vi "OTF_subtraction.vi"(0 "Buffer Length":i32, 5 "Buffer":u32[](array[numeric]), 7 "Cluster In":T1 {"Coincidence Window" format="%#_13g"; "Delay12" format="%#_13g"; "Delay02" format="%#_13g"; "Delay01" format="%#_13g"}, 12 "ofl":u64) -> (3 "ofl out":u64, 8 "output cluster":T1 {"Coincidence Window" format="%#_13g"; "Delay12" format="%#_13g"; "Delay02" format="%#_13g"; "Delay01" format="%#_13g"})   [LabVIEW 2023]
uses:
  Get_Delays_Ctrl.ctl
panel:
  out "Delay02":dbl
  out "Delay12":dbl
  out "Trues":dbl
  out "Delay01":dbl
  out "Coincidence Triggers":u64
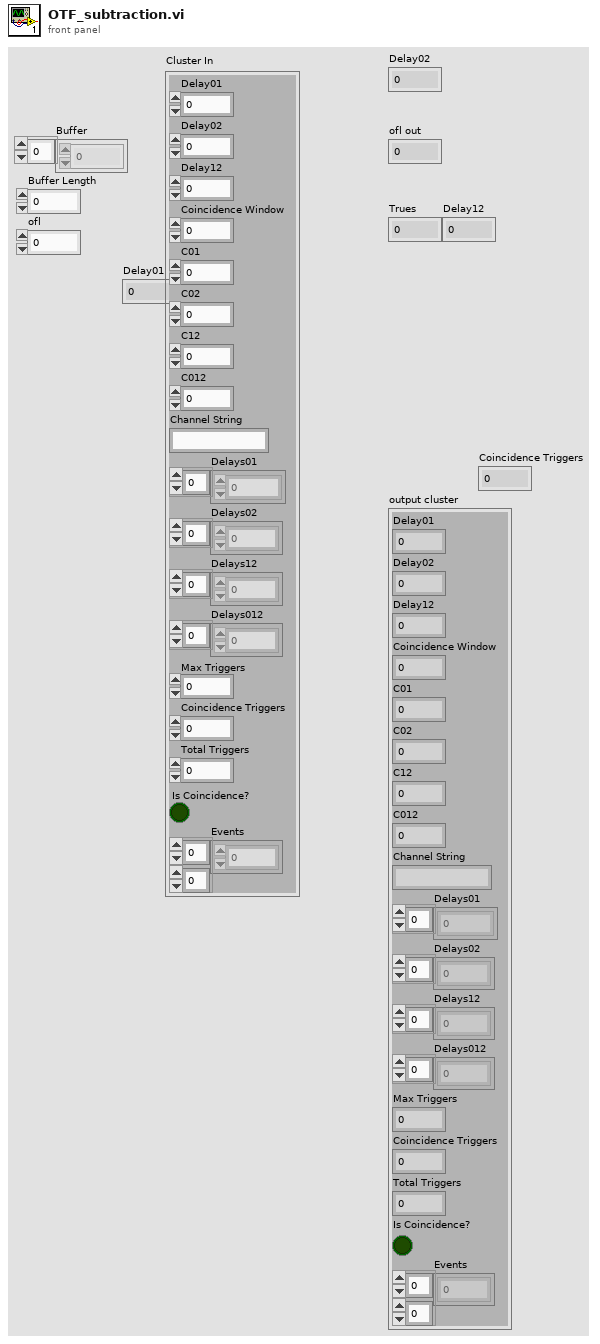
[diagram p1: front panel]
types:
  T1 = typedef "Get_Delays_Ctrl.ctl" = cluster{"Delay01":dbl, "Delay02":dbl, "Delay12":dbl, "Coincidence Window":dbl, "C01":u32, "C02":u32, "C12":u32, "C012":u32, "Channel String":string, "Delays01":sgl[], "Delays02":dbl[], "Delays12":dbl[], "Delays012":dbl[], "Max Triggers":i32, "Coincidence Triggers":i32, "Total Triggers":i32, "Is Coincidence?":bool, "Events":u64[][]}
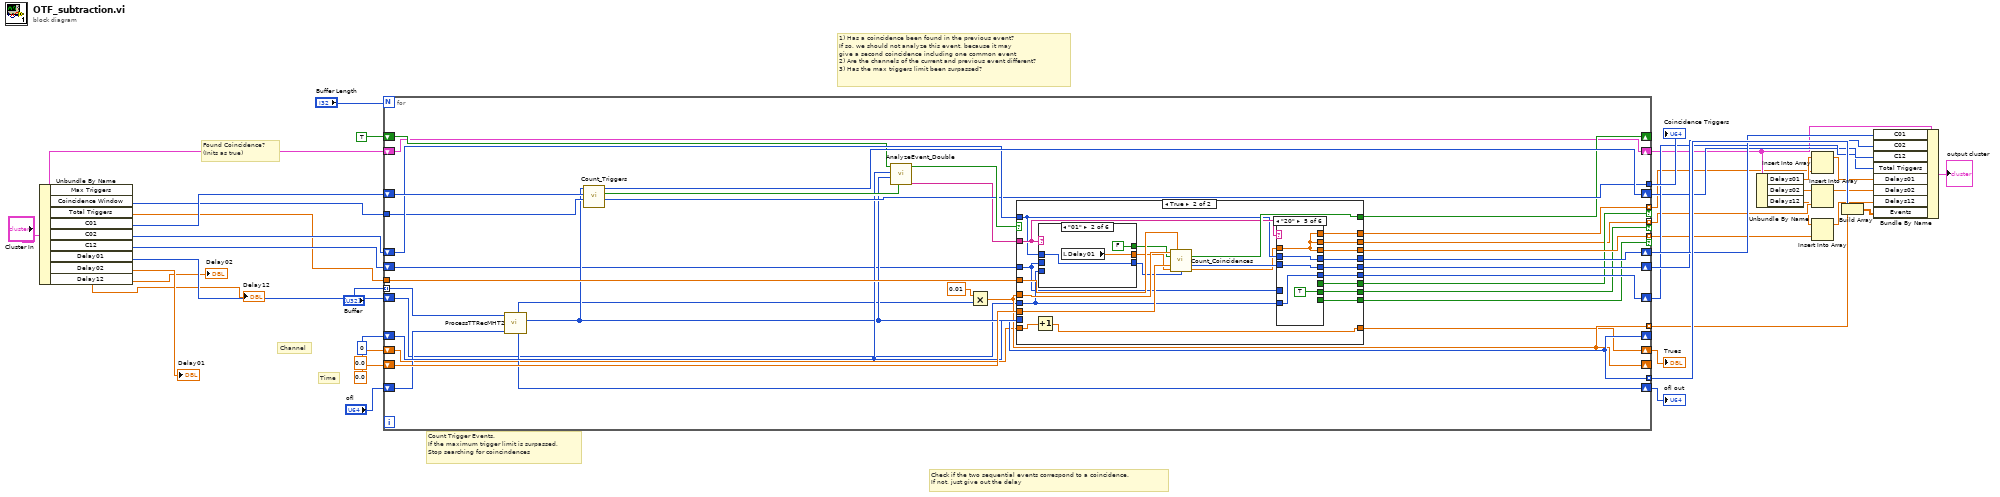
[diagram p0: block diagram]
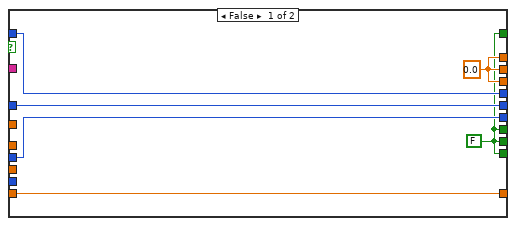
[diagram p2: hidden frame]
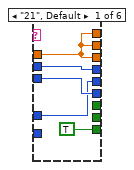
[diagram p3: hidden frame]
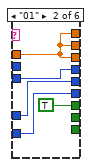
[diagram p4: hidden frame]
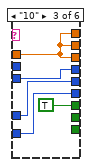
[diagram p5: hidden frame]
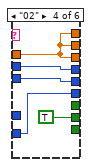
[diagram p6: hidden frame]
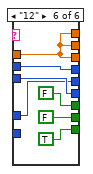
[diagram p7: hidden frame]
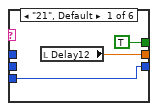
[diagram p8: hidden frame]
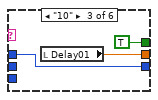
[diagram p9: hidden frame]
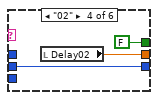
[diagram p10: hidden frame]
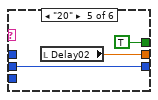
[diagram p11: hidden frame]
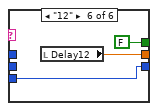
[diagram p12: hidden frame]
diagram:
  # "Count Trigger Events.\nIf the maximum trigger limit is surpassed,\nStop searching for coincindences"
  # "Check if the two sequential events correspond to a coincidence. \nIf not, just give out the delay"
  # "1) Has a coincidence been found in the previous event? \nIf so, we should not analyze this event, because it may\ngive a second coincidence including one common event\n2) Are the channels of the current and previous event different?\n3) Has the max triggers limit been surpassed?"
  # "Found Coincidence?\n(Inits as true)"
  # "Time"
  # "Channel"
  n1 = Unbundle By Name("Cluster In") -> ("Max Triggers"=w14:i32, "Coincidence Window"=w15:dbl, "Total Triggers"=w25:i32, "C01"=w18:u32, "C02"=w17:u32, "C12"=w16:u32, "Delay01"=→"Delay01":dbl, "Delay02"=→"Delay02":dbl, "Delay12"=→"Delay12":dbl)
  n2 = for {
    N: "Buffer Length" -> [_]
    shift-right: [w54] -> _
    shift-left: 0.0 ("number: 0 to 1") -> [w69]
    tunnel: [w45] -> w8 mode=indexing if=w43
    shift-right: [w59] -> _
    shift-left: u32 0 ("number") -> [w61]
    tunnel: [w59] -> w30 mode=indexing
    tunnel: [w54] -> w29 mode=indexing
    shift-right: [w71] -> w20
    shift-left: w25 -> [w72]
    shift-right: [w68] -> w23
    shift-left: w18 -> [w70]
    shift-right: [w60] -> _
    shift-left: TRUE ("Is Coincidence?") -> [w66]
    tunnel: [w65] -> w35
    tunnel: w14 -> [w63]
    tunnel: w15 -> [w62]
    tunnel: "Buffer" -> [w58] mode=indexing
    shift-right: [w56] -> w31
    shift-left: "ofl" -> [w57]
    shift-right: [w52] -> w27
    shift-left: 0.0 -> [w51]
    shift-right: [w47] -> w21
    shift-left: w16 -> [w49]
    shift-right: [w46] -> w22
    shift-left: w17 -> [w48]
    tunnel: [w44] -> w3 mode=indexing if=w41
    tunnel: [w42] -> w4 mode=indexing if=w40
    shift-right: [w39] -> w10
    shift-left: "Cluster In" -> [w39]
    n3 = call "ProcessTTRecMHT2.vi"("oflcorr_in"=w57, "rawbits"=w58) -> ("channel"=w59:u32, "oflcorr_out"=w56:u64, "timetag"=w55:u64)  [unwired: 4 in, 3 out]
    n4 = call "Count_Triggers.vi"("Max Triggers"=w63, "Triggers In"=w72, "channel"=w59) -> ("Coincidence Triggers"=w65:u64, "Max triggers?"=w64:bool, "Total Triggers Out"=w71:u64)  [unwired: 6 in]
    n5 = call "AnalyzeEvent_Double.vi"("Max triggers?"=w64, "Channel - Current"=w59, "Channel - Previous"=w61, "Is Coincidence?"=w66) -> ("Coincidence Type"=w50:string, "Analyze?"=w67:bool)  [unwired: 6 in]
    n6 = Multiply(x=0.01, y=w55) -> (x*y=w54:dbl)
    n7 = case shown="True" w67 {
      tunnel: w70 -> [w78 w88]
      tunnel: w62 -> [_ w102]
      tunnel: w69 -> [_ w101]
      tunnel: w61 -> [_ _]
      tunnel: w54 -> [_ w100]
      tunnel: [w73 w99] -> w60
      tunnel: [w78 w89] -> w68
      tunnel: [w73 w84] -> w43
      tunnel: w51 -> [w77 w98]
      tunnel: [w77 w97] -> w52
      tunnel: w50 -> [_ w93]
      tunnel: w49 -> [w75 w87]
      tunnel: w48 -> [w76 w86]
      tunnel: [w75 w91] -> w47
      tunnel: [w76 w90] -> w46
      tunnel: [w74 w85] -> w45
      tunnel: [w74 w83] -> w44
      tunnel: [w74 w82] -> w42
      tunnel: [w73 w81] -> w41
      tunnel: [w73 w80] -> w40
      frame False {
        w74 = 0.0 ("Delay")
        w73 = FALSE ("Is Coincidence?")
      }
      frame True {
        n8 = Increment(x=w98) -> (x+1=w97:dbl)
        n9 = case shown="\"01\"" w93 {
          tunnel: [w135 w140 w143 w144 w147 w150] -> w96
          tunnel: w88 -> [_ w140 w143 _ _ _]
          tunnel: [w136 w139 w142 w146 w149 w152] -> w95
          tunnel: [TRUE ("Is Coincidence?") FALSE ("Is Coincidence?") TRUE ("Is Coincidence?") FALSE ("Is Coincidence?") TRUE ("Is Coincidence?") FALSE ("Is Coincidence?")] -> w94
          tunnel: w87 -> [w135 _ _ _ _ w150]
          tunnel: w86 -> [_ _ _ w144 w147 _]
          frame "21", Default {
            n10 = local read "Delay12"() -> (w136:dbl)
          }
          frame "01" {
            n11 = local read "Delay01"() -> (w139:dbl)
          }
          frame "10" {
            n12 = local read "Delay01"() -> (w142:dbl)
          }
          frame "02" {
            n13 = local read "Delay02"() -> (w146:dbl)
          }
          frame "20" {
            n14 = local read "Delay02"() -> (w149:dbl)
          }
          frame "12" {
            n15 = local read "Delay12"() -> (w152:dbl)
          }
        }
        n16 = call "Count_Coincidences.vi"("Time-Current"=w100, "Coincidence Window"=w102, "Reverse?"=w94, "Time - Previous"=w101, "Expected Delay"=w95, "Coincidences In"=w96) -> ("Is Coincidence?"=w99:bool, "Coincidences Out"=w92:u32, "Shifted Delay"=w79:dbl)  [unwired: 6 in, 1 out]
        n17 = case shown="\"20\"" w93 {
          tunnel: [w107 w111 w115 w120 w127 w134] -> w91
          tunnel: w92 -> [w107 w112 w117 w122 w125 w134]
          tunnel: [w105 w110 w116 w122 w125 w133] -> w90
          tunnel: [w106 w112 w117 w121 w126 w132] -> w89
          tunnel: w88 -> [w106 _ _ w121 w126 w132]
          tunnel: w87 -> [_ w111 w115 w120 w127 _]
          tunnel: w86 -> [w105 w110 w116 _ _ w133]
          tunnel: [w104 w108 w113 w119 w124 w131] -> w85
          tunnel: w79 -> [w104 w108 w113 w119 w124 w131]
          tunnel: [_ TRUE ("Is Coincidence?") TRUE ("Is Coincidence?") _ _ FALSE ("Is Coincidence?")] -> w84
          tunnel: [w104 w108 w113 w119 w124 w131] -> w83
          tunnel: [w104 w108 w113 w119 w124 w131] -> w82
          tunnel: [TRUE ("Is Coincidence?") _ _ _ _ TRUE ("Is Coincidence?")] -> w81
          tunnel: [_ _ _ TRUE ("Is Coincidence?") TRUE ("Is Coincidence?") FALSE ("Is Coincidence?")] -> w80
          frame "21", Default {
          }
          frame "01" {
          }
          frame "10" {
          }
          frame "02" {
          }
          frame "20" {
          }
          frame "12" {
          }
        }
      }
    }
  }
  "Coincidence Triggers" <- w35
  "ofl out" <- w31
  "Trues" <- w27
  n18 = Unbundle By Name(w10) -> ("Delays01"=w9:sgl[], "Delays02"=w5:dbl[], "Delays12"=w1:dbl[])
  n19 = Insert Into Array(array=w9, new element=w8) -> (w7:sgl[])  [unwired: 1 in]
  n20 = Insert Into Array(array=w5, new element=w4) -> (w6:dbl[])  [unwired: 1 in]
  n21 = Insert Into Array(array=w1, new element=w3) -> (w2:dbl[])  [unwired: 1 in]
  n22 = Build Array(w30, w29) -> (w19:dbl[][])
  n23 = Bundle By Name(cluster=w10, "C01"=w23, "C02"=w22, "C12"=w21, "Total Triggers"=w20, "Delays01"=w7, "Delays02"=w6, "Delays12"=w2, "Events"=w19) -> (→"output cluster":T1)
